vi "GetType.vi"(8 "error in (no error)":errorcluster, 11 "Polling Start Stop Msg":refnum<class "Polling Start Stop Msg.lvclass">) -> (0 "error out":errorcluster, 2 "Data Sample":variant, 3 "Polling Start Stop Msg":refnum<class "Polling Start Stop Msg.lvclass">)   [LabVIEW 2015, in "CS++BaseActor.lvlib" / "Polling Start Stop Msg.lvclass"]
uses:
  Polling Start Stop Msg.lvclass
  Polling Start Stop Msg.lvclass/Polling Start Stop Msg.ctl
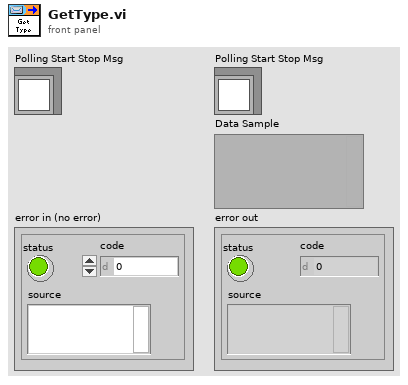
[diagram p1: front panel]
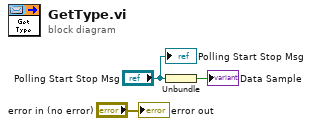
[diagram p0: block diagram]
diagram:
  n1 = Unbundle("Polling Start Stop Msg") -> (→"Data Sample":bool)
  "error out" <- "error in (no error)"
  "Polling Start Stop Msg" <- "Polling Start Stop Msg"
